vi "String to level meter device cluster.vi"(11 "LVL Device Details":string="STAT:40000000:NIT:FREQ:ZERO:0:FULL:0:PPS:750:MAN:HVER:1:FVER:1.8:SERL:111450013:HEL:RES:ZERO:0:FULL:0:PULS:TIM::DEL:0:MAG:0:PREP:TIM:0:MAG:0:SIG:NIT:COUN:0.0000n:FREQ:0:LEV:0.0000%:HEL:LEV:0.0000%:RES:0.0000O") -> (3 "Level Meter":T1)   [LabVIEW 2019, in "Mercury iXX.lvlib" / "Level Meter.lvlib"]
uses:
  Level Meter.lvlib
  Controls/Level Meter (Read).ctl
  Controls/Manufacturing Data.ctl
  Controls/Nitrogen Configuration.ctl
  Controls/Frequency Configuration.ctl
  Controls/Signals.ctl
  Controls/Helium Configuration.ctl
  Controls/Resistance Configuration.ctl
  Controls/Pre-Pulse.ctl
  Controls/Pulse.ctl
  mercury/Mercury iXX.lvlib
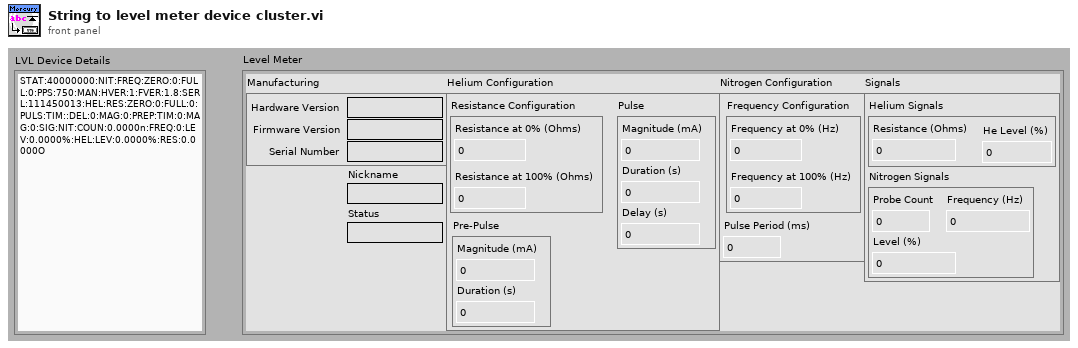
[diagram p1: front panel]
types:
  T1 = typedef "Mercury iXX.lvlib/Level Meter.lvlib/Level Meter (Read).ctl" = cluster{"Manufacturing":T2, "Nitrogen Configuration":T3, "Signals":T5, "Nickname":string, "Status":string, "Helium Configuration":T6}
  T2 = typedef "Mercury iXX.lvlib/Manufacturing Data.ctl" = cluster{"Hardware Version":string, "Firmware Version":string, "Serial Number":string}
  T3 = typedef "Mercury iXX.lvlib/Level Meter.lvlib/Nitrogen Configuration.ctl" = cluster{"Frequency Configuration":T4, "Pulse Period":dbl}
  T4 = typedef "Mercury iXX.lvlib/Level Meter.lvlib/Frequency Configuration.ctl" = cluster{"Freq 0%":dbl, "Freq 100%":dbl}
  T5 = typedef "Mercury iXX.lvlib/Level Meter.lvlib/Signals.ctl" = cluster{"Helium Signals":cluster{"Resistance":dbl, "Level":dbl}, "Nitrogen Signals":cluster{"Count":dbl, "Freq":dbl, "Level":dbl}}
  T6 = typedef "Mercury iXX.lvlib/Level Meter.lvlib/Helium Configuration.ctl" = cluster{"Resistance Configuration":T7, "Pre-Pulse":T8, "Pulse":T9}
  T7 = typedef "Mercury iXX.lvlib/Level Meter.lvlib/Resistance Configuration.ctl" = cluster{"Res 0%":dbl, "Res 100%":dbl}
  T8 = typedef "Mercury iXX.lvlib/Level Meter.lvlib/Pre-Pulse.ctl" = cluster{"Magnitude":dbl, "Duration":dbl}
  T9 = typedef "Mercury iXX.lvlib/Level Meter.lvlib/Pulse.ctl" = cluster{"Magnitude":dbl, "Duration":dbl, "Delay":dbl}
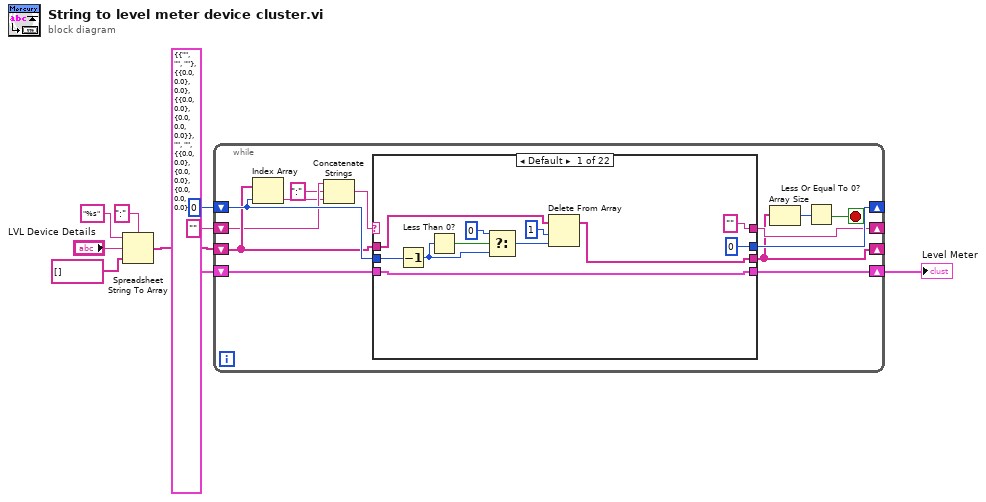
[diagram p0: block diagram]
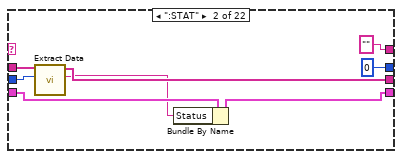
[diagram p2: hidden frame]
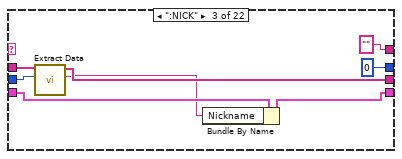
[diagram p3: hidden frame]
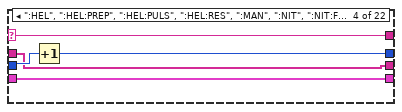
[diagram p4: hidden frame]
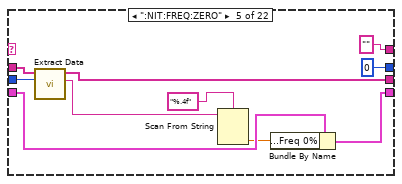
[diagram p5: hidden frame]
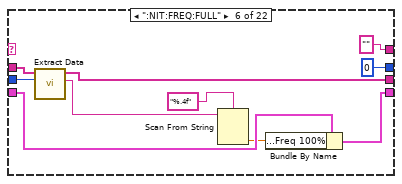
[diagram p6: hidden frame]
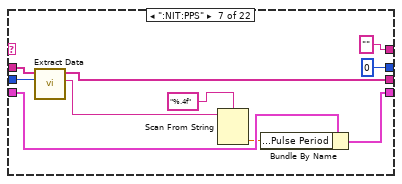
[diagram p7: hidden frame]
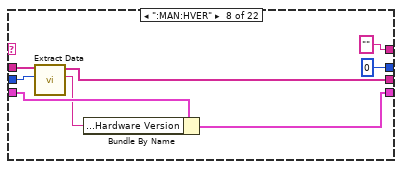
[diagram p8: hidden frame]
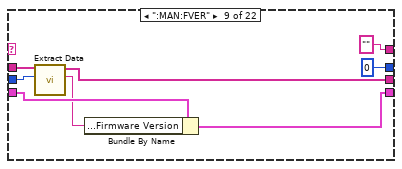
[diagram p9: hidden frame]
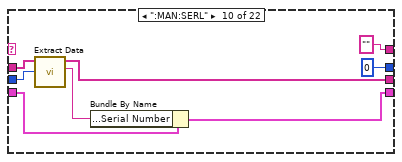
[diagram p10: hidden frame]
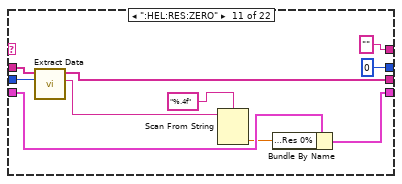
[diagram p11: hidden frame]
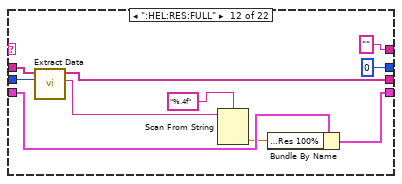
[diagram p12: hidden frame]
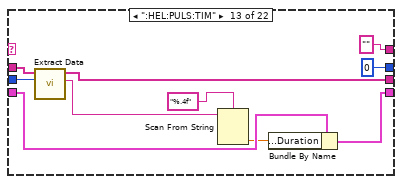
[diagram p13: hidden frame]
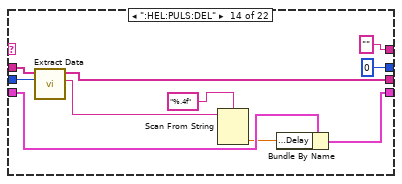
[diagram p14: hidden frame]
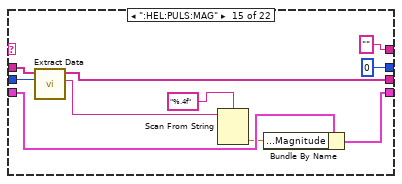
[diagram p15: hidden frame]
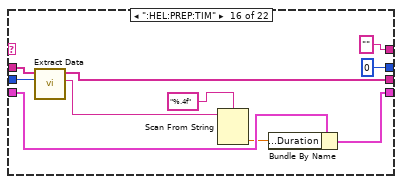
[diagram p16: hidden frame]
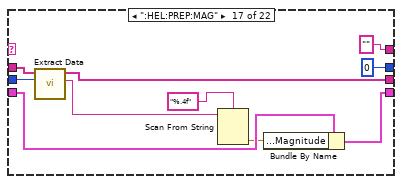
[diagram p17: hidden frame]
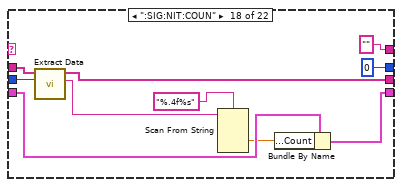
[diagram p18: hidden frame]
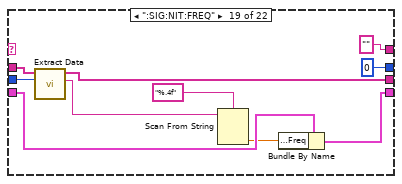
[diagram p19: hidden frame]
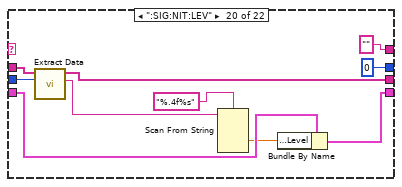
[diagram p20: hidden frame]
diagram:
  n1 = Spreadsheet String To Array(delimiter (Tab)=":", format string="%s", spreadsheet string="LVL Device Details", array type (2D Dbl)=string[] []) -> (array=w4:string[])
  n2 = while {
    shift-right: [w20] -> _
    shift-left: 0 ("index") -> [w22]
    shift-right: [w18] -> _
    shift-left: "" -> [w19]
    shift-right: [w12] -> _
    shift-left: w4 -> [w21]
    shift-right: [w10] -> w1
    shift-left: T1 {"Manufacturing"={"Hardware Version"="", "Firmware Version"="", "Serial Number"=""}, "Nitrogen Configuration"={"Frequency Configuration"={"Freq 0%"=0.0, "Freq 100%"=0.0}, "Pulse Period"=0.0}, "Signals"={"Helium Signals"={"Resistance"=0.0, "Level"=0.0}, "Nitrogen Signals"={"Count"=0.0, "Freq"=0.0, "Level"=0.0}}, "Nickname"="", "Status"="", "Helium Configuration"={"Resistance Configuration"={"Res 0%"=0.0, "Res 100%"=0.0}, "Pre-Pulse"={"Magnitude"=0.0, "Duration"=0.0}, "Pulse"={"Magnitude"=0.0, "Duration"=0.0, "Delay"=0.0}}} ("Level Meter") -> [w11]
    stop <- w14 stop-if-true
    n3 = Index Array(array=w21, index=w22) -> (element=w17:string)
    n4 = Concatenate Strings(w19, ":" ("string"), w17) -> (w13:string)
    n5 = case shown="Default" w13 {
      selector: w13 -> [_ _ _ w54 _ _ _ _ _ _ _ _ _ _ _ _ _ _ _ _ _ _]
      tunnel: w22 -> [w33 w37 w48 w53 w60 w73 w83 w91 w99 w106 w116 w126 w136 w147 w157 w167 w177 w187 w197 w207 w216 w225]
      tunnel: w21 -> [w31 w39 w49 w51 w62 w74 w84 w92 w100 w108 w118 w128 w138 w148 w158 w168 w178 w188 w198 w208 w217 w226]
      tunnel: [0 ("index") 0 ("index") 0 ("index") w52 0 ("index") 0 ("index") 0 ("index") 0 ("index") 0 ("index") 0 ("index") 0 ("index") 0 ("index") 0 ("index") 0 ("index") 0 ("index") 0 ("index") 0 ("index") 0 ("index") 0 ("index") 0 ("index") 0 ("index") 0 ("index")] -> w20
      tunnel: ["" "" "" w54 "" "" "" "" ("Data") "" ("Data") "" ("Data") "" ("Data") "" ("Data") "" ("Data") "" ("Data") "" ("Data") "" ("Data") "" ("Data") "" ("Data") "" ("Data") "" ("Data") "" ""] -> w18
      tunnel: [w30 w38 w47 w51 w61 w72 w82 w90 w98 w107 w117 w127 w137 w146 w156 w166 w176 w186 w196 w206 w218 w224] -> w12
      tunnel: w11 -> [w27 w36 w44 w50 w59 w69 w79 w87 w95 w103 w113 w123 w133 w143 w153 w163 w173 w183 w193 w203 w213 w223]
      tunnel: [w27 w35 w43 w50 w58 w68 w77 w86 w94 w102 w111 w121 w131 w141 w151 w161 w171 w182 w192 w200 w210 w220] -> w10
      frame Default {
        n6 = Decrement(x=w33) -> (x-1=w25:i32)
        n7 = Less Than 0?(x=w25) -> (x < 0?=w26:bool)
        n8 = Select(t=0, s=w26, f=w25) -> (s? t:f=w23:i32)
        n9 = Delete From Array(array=w31, length=1, index=w23) -> (array with subset deleted=w30:string[])  [unwired: 1 out]
      }
      frame ":STAT" {
        n10 = call "Extract Data.vi"("index in"=w37, "Array In"=w39) -> ("Data"=w34:string, "Array Out"=w38:string[])  [unwired: 8 out]
        n11 = Bundle By Name(cluster=w36, "Status"=w34) -> (w35:T1)
      }
      frame ":NICK" {
        n12 = call "Extract Data.vi"("index in"=w48, "Array In"=w49) -> ("Data"=w42:string, "Array Out"=w47:string[])  [unwired: 8 out]
        n13 = Bundle By Name(cluster=w44, "Nickname"=w42) -> (w43:T1)
      }
      frame ":HEL", ":HEL:PREP", ":HEL:PULS", ":HEL:RES", ":MAN", ":NIT", ":NIT:FREQ", ":SIG", ":SIG:HEL", ":SIG:NIT" {
        n14 = Increment(x=w53) -> (x+1=w52:i32)
      }
      frame ":NIT:FREQ:ZERO" {
        n15 = call "Extract Data.vi"("index in"=w60, "Array In"=w62) -> ("Data"=w56:string, "Array Out"=w61:string[])  [unwired: 8 out]
        n16 = Scan From String(format string="%.4f", input string=w56) -> (output 1=w55:dbl)  [unwired: 2 in, 4 out]
        n17 = Bundle By Name(cluster=w59, "Nitrogen Configuration.Frequency Configuration.Freq 0%"=w55) -> (w58:T1)
      }
      frame ":NIT:FREQ:FULL" {
        n18 = call "Extract Data.vi"("index in"=w73, "Array In"=w74) -> ("Data"=w66:string, "Array Out"=w72:string[])  [unwired: 1 in, 7 out]
        n19 = Scan From String(format string="%.4f", input string=w66) -> (output 1=w65:dbl)  [unwired: 2 in, 4 out]
        n20 = Bundle By Name(cluster=w69, "Nitrogen Configuration.Frequency Configuration.Freq 100%"=w65) -> (w68:T1)
      }
      frame ":NIT:PPS" {
        n21 = call "Extract Data.vi"("index in"=w83, "Array In"=w84) -> ("Data"=w75:string, "Array Out"=w82:string[])  [unwired: 8 out]
        n22 = Scan From String(format string="%.4f", input string=w75) -> (output 1=w76:dbl)  [unwired: 2 in, 4 out]
        n23 = Bundle By Name(cluster=w79, "Nitrogen Configuration.Pulse Period"=w76) -> (w77:T1)
      }
      frame ":MAN:HVER" {
        n24 = call "Extract Data.vi"("index in"=w91, "Array In"=w92) -> ("Data"=w85:string, "Array Out"=w90:string[])  [unwired: 8 out]
        n25 = Bundle By Name(cluster=w87, "Manufacturing.Hardware Version"=w85) -> (w86:T1)
      }
      frame ":MAN:FVER" {
        n26 = call "Extract Data.vi"("index in"=w99, "Array In"=w100) -> ("Data"=w93:string, "Array Out"=w98:string[])  [unwired: 8 out]
        n27 = Bundle By Name(cluster=w95, "Manufacturing.Firmware Version"=w93) -> (w94:T1)
      }
      frame ":MAN:SERL" {
        n28 = call "Extract Data.vi"("index in"=w106, "Array In"=w108) -> ("Data"=w101:string, "Array Out"=w107:string[])  [unwired: 8 out]
        n29 = Bundle By Name(cluster=w103, "Manufacturing.Serial Number"=w101) -> (w102:T1)
      }
      frame ":HEL:RES:ZERO" {
        n30 = call "Extract Data.vi"("index in"=w116, "Array In"=w118) -> ("Data"=w109:string, "Array Out"=w117:string[])  [unwired: 8 out]
        n31 = Scan From String(format string="%.4f", input string=w109) -> (output 1=w110:dbl)  [unwired: 2 in, 4 out]
        n32 = Bundle By Name(cluster=w113, "Helium Configuration.Resistance Configuration.Res 0%"=w110) -> (w111:T1)
      }
      frame ":HEL:RES:FULL" {
        n33 = call "Extract Data.vi"("index in"=w126, "Array In"=w128) -> ("Data"=w119:string, "Array Out"=w127:string[])  [unwired: 8 out]
        n34 = Scan From String(format string="%.4f", input string=w119) -> (output 1=w120:dbl)  [unwired: 2 in, 4 out]
        n35 = Bundle By Name(cluster=w123, "Helium Configuration.Resistance Configuration.Res 100%"=w120) -> (w121:T1)
      }
      frame ":HEL:PULS:TIM" {
        n36 = call "Extract Data.vi"("index in"=w136, "Array In"=w138) -> ("Data"=w129:string, "Array Out"=w137:string[])  [unwired: 8 out]
        n37 = Scan From String(format string="%.4f", input string=w129) -> (output 1=w130:dbl)  [unwired: 2 in, 4 out]
        n38 = Bundle By Name(cluster=w133, "Helium Configuration.Pulse.Duration"=w130) -> (w131:T1)
      }
      frame ":HEL:PULS:DEL" {
        n39 = call "Extract Data.vi"("index in"=w147, "Array In"=w148) -> ("Data"=w139:string, "Array Out"=w146:string[])  [unwired: 8 out]
        n40 = Scan From String(format string="%.4f", input string=w139) -> (output 1=w140:dbl)  [unwired: 2 in, 4 out]
        n41 = Bundle By Name(cluster=w143, "Helium Configuration.Pulse.Delay"=w140) -> (w141:T1)
      }
      frame ":HEL:PULS:MAG" {
        n42 = call "Extract Data.vi"("index in"=w157, "Array In"=w158) -> ("Data"=w149:string, "Array Out"=w156:string[])  [unwired: 8 out]
        n43 = Scan From String(format string="%.4f", input string=w149) -> (output 1=w150:dbl)  [unwired: 2 in, 4 out]
        n44 = Bundle By Name(cluster=w153, "Helium Configuration.Pulse.Magnitude"=w150) -> (w151:T1)
      }
      frame ":HEL:PREP:TIM" {
        n45 = call "Extract Data.vi"("index in"=w167, "Array In"=w168) -> ("Data"=w159:string, "Array Out"=w166:string[])  [unwired: 8 out]
        n46 = Scan From String(format string="%.4f", input string=w159) -> (output 1=w160:dbl)  [unwired: 2 in, 4 out]
        n47 = Bundle By Name(cluster=w163, "Helium Configuration.Pre-Pulse.Duration"=w160) -> (w161:T1)
      }
      frame ":HEL:PREP:MAG" {
        n48 = call "Extract Data.vi"("index in"=w177, "Array In"=w178) -> ("Data"=w169:string, "Array Out"=w176:string[])  [unwired: 8 out]
        n49 = Scan From String(format string="%.4f", input string=w169) -> (output 1=w170:dbl)  [unwired: 2 in, 4 out]
        n50 = Bundle By Name(cluster=w173, "Helium Configuration.Pre-Pulse.Magnitude"=w170) -> (w171:T1)
      }
      frame ":SIG:NIT:COUN" {
        n51 = call "Extract Data.vi"("index in"=w187, "Array In"=w188) -> ("Data"=w180:string, "Array Out"=w186:string[])  [unwired: 8 out]
        n52 = Scan From String(format string="%.4f%s", input string=w180) -> (output 1=w179:dbl)  [unwired: 2 in, 6 out]
        n53 = Bundle By Name(cluster=w183, "Signals.Nitrogen Signals.Count"=w179) -> (w182:T1)
      }
      frame ":SIG:NIT:FREQ" {
        n54 = call "Extract Data.vi"("index in"=w197, "Array In"=w198) -> ("Data"=w190:string, "Array Out"=w196:string[])  [unwired: 8 out]
        n55 = Scan From String(format string="%.4f", input string=w190) -> (output 1=w191:dbl)  [unwired: 2 in, 4 out]
        n56 = Bundle By Name(cluster=w193, "Signals.Nitrogen Signals.Freq"=w191) -> (w192:T1)
      }
      frame ":SIG:NIT:LEV" {
        n57 = call "Extract Data.vi"("index in"=w207, "Array In"=w208) -> ("Data"=w201:string, "Array Out"=w206:string[])  [unwired: 8 out]
        n58 = Scan From String(format string="%.4f%s", input string=w201) -> (output 1=w199:dbl)  [unwired: 2 in, 6 out]
        n59 = Bundle By Name(cluster=w203, "Signals.Nitrogen Signals.Level"=w199) -> (w200:T1)
      }
      frame ":SIG:HEL:LEV" {
        n60 = call "Extract Data.vi"("index in"=w216, "Array In"=w217) -> ("Data"=w211:string, "Array Out"=w218:string[])  [unwired: 8 out]
        n61 = Scan From String(format string="%.4f%s", input string=w211) -> (output 1=w209:dbl)  [unwired: 2 in, 6 out]
        n62 = Bundle By Name(cluster=w213, "Signals.Helium Signals.Level"=w209) -> (w210:T1)
      }
      frame ":SIG:HEL:RES" {
        n63 = call "Extract Data.vi"("index in"=w225, "Array In"=w226) -> ("Data"=w221:string, "Array Out"=w224:string[])  [unwired: 8 out]
        n64 = Scan From String(format string="%.4f%s", input string=w221) -> (output 1=w219:dbl)  [unwired: 2 in, 6 out]
        n65 = Bundle By Name(cluster=w223, "Signals.Helium Signals.Resistance"=w219) -> (w220:T1)
      }
    }
    n66 = Array Size(array=w12) -> (size(s)=w15:i32)
    n67 = Less Or Equal To 0?(x=w15) -> (x <= 0?=w14:bool)
  }
  "Level Meter" <- w1
